vi "LoadAdditionalData.vi"(8 "error in (no error)":errorcluster, 11 "TesteractHAL_DigitalOutput_NIDAQmx In":refnum<class "TesteractHAL_DigitalOutput_NIDAQmx.lvclass">) -> (0 "error out":errorcluster, 3 "TesteractHAL_DigitalOutput_NIDAQmx Out":refnum<class "TesteractHAL_DigitalOutput_NIDAQmx.lvclass">)   [LabVIEW 2017, in "TesteractHAL_DigitalOutput_NIDAQmx.lvlib" / "TesteractHAL_DigitalOutput_NIDAQmx.lvclass"]
doc: "Reads all the data from DeviceCfg and uploads it into the class private data."
uses:
  TesteractHAL_DigitalOutput_NIDAQmx.lvclass
  C:/Program Files (x86)/Testeract/HWLib/HAL/Device/TesteractHAL_Device.lvlibp/TesteractHAL_Device.lvclass
  TesteractHAL_DigitalOutput_NIDAQmx.lvclass/TesteractHAL_DigitalOutput_NIDAQmx.ctl
  Program Files (x86)/Testeract/HWLib/HAL/Device/TesteractHAL_Device.lvlibp/ReadDeviceName.vi
  Program Files (x86)/Testeract/HWLib/HAL/DeviceCfg/TesteractHAL_DeviceCfg_API.lvlibp
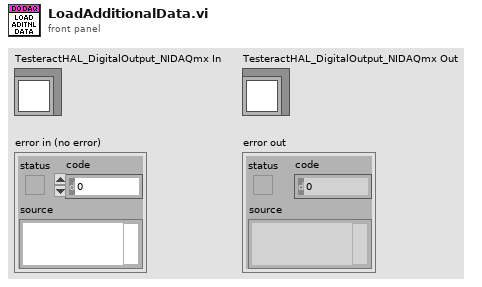
[diagram p1: front panel]
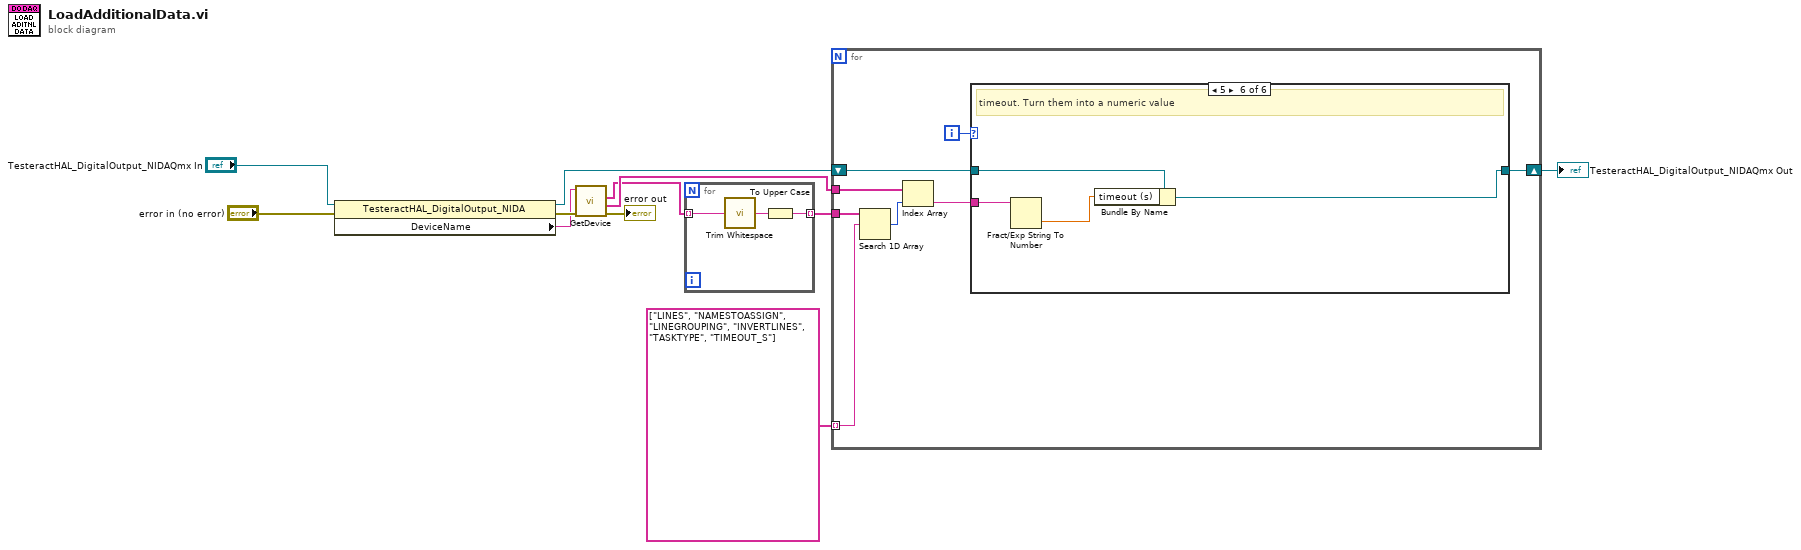
[diagram p0: block diagram]
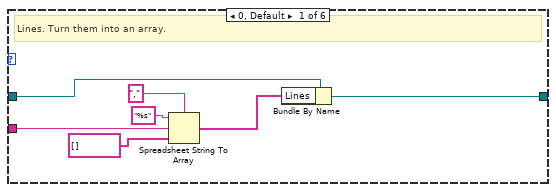
[diagram p2: hidden frame]
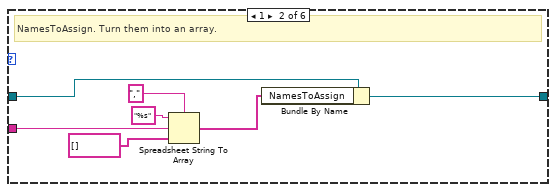
[diagram p3: hidden frame]
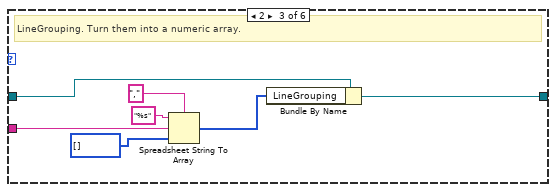
[diagram p4: hidden frame]
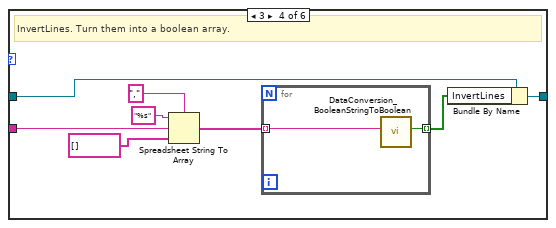
[diagram p5: hidden frame]
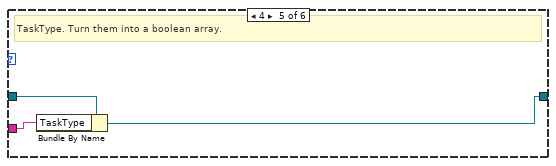
[diagram p6: hidden frame]
diagram:
  n1 = property class="TesteractHAL_DigitalOutput_NIDA"(reference="TesteractHAL_DigitalOutput_NIDAQmx In", error in="error in (no error)") -> (reference out=w2:refnum<class "TesteractHAL_DigitalOutput_NIDAQmx.lvclass">, error out=w9:errorcluster, "DeviceName"=w8:string)
  n2 = call "GetDevice.vi"("error in (no error)"=w9, "Device"=w8) -> ("error out"=→"error out":errorcluster, "Values"=w7:string[], "Keys"=w4:string[])  [unwired: 6 in, 1 out]
  n3 = for {
    tunnel: [w14] -> w5 mode=indexing
    tunnel: w4 -> [w13] mode=indexing
    n4 = call <vilib>:"Trim Whitespace.vi"("string"=w13) -> ("trimmed string"=w12:string)  [unwired: 1 in]
    n5 = To Upper Case(1:w12) -> (0:w14:string)
  }
  n6 = for {
    tunnel: w7 -> [w16]
    tunnel: string[] ["LINES", "NAMESTOASSIGN", "LINEGROUPING", "INVERTLINES", "TASKTYPE", "TIMEOUT_S"] -> [w18] mode=indexing
    tunnel: w5 -> [w17]
    shift-right: [w19] -> w1
    shift-left: w2 -> [w20]
    i -> [w22]
    n7 = Search 1D Array(1D array=w17, element=w18) -> (index of element=w21:i32)  [unwired: 1 in]
    n8 = Index Array(array=w16, index=w21) -> (element=w15:string)
    n9 = case shown="5" w22 {
      tunnel: w20 -> [w29 w35 w42 w50 w55 w59]
      tunnel: [w28 w36 w43 w51 w56 w60] -> w19
      tunnel: w15 -> [w24 w31 w38 w46 w54 w58]
      frame 0, Default {
        # "Lines. Turn them into an array."
        n10 = Spreadsheet String To Array(delimiter (Tab)=",", format string="%s", spreadsheet string=w24, array type (2D Dbl)=string[] []) -> (array=w23:string[])
        n11 = Bundle By Name(cluster=w29, "Lines"=w23) -> (w28:refnum<class "TesteractHAL_DigitalOutput_NIDAQmx.lvclass">)
      }
      frame 1 {
        # "NamesToAssign. Turn them into an array."
        n12 = Spreadsheet String To Array(delimiter (Tab)=",", format string="%s", spreadsheet string=w31, array type (2D Dbl)=string[] []) -> (array=w30:string[])
        n13 = Bundle By Name(cluster=w35, "NamesToAssign"=w30) -> (w36:refnum<class "TesteractHAL_DigitalOutput_NIDAQmx.lvclass">)
      }
      frame 2 {
        # "LineGrouping. Turn them into a numeric array."
        n14 = Spreadsheet String To Array(delimiter (Tab)=",", format string="%s", spreadsheet string=w38, array type (2D Dbl)=i32[] [] ("LineGrouping")) -> (array=w37:i32[])
        n15 = Bundle By Name(cluster=w42, "LineGrouping"=w37) -> (w43:refnum<class "TesteractHAL_DigitalOutput_NIDAQmx.lvclass">)
      }
      frame 3 {
        # "InvertLines. Turn them into a boolean array."
        n16 = Spreadsheet String To Array(delimiter (Tab)=",", format string="%s", spreadsheet string=w46, array type (2D Dbl)=string[] []) -> (array=w45:string[])
        n17 = for {
          tunnel: w45 -> [w53] mode=indexing
          tunnel: [w52] -> w44 mode=indexing
          n18 = call "DataConversion_BooleanStringToBoolean.vi"("Boolean String"=w53) -> ("Boolean Result"=w52:bool)  [unwired: 10 in]
        }
        n19 = Bundle By Name(cluster=w50, "InvertLines"=w44) -> (w51:refnum<class "TesteractHAL_DigitalOutput_NIDAQmx.lvclass">)
      }
      frame 4 {
        # "TaskType. Turn them into a boolean array."
        n20 = Bundle By Name(cluster=w55, "TaskType"=w54) -> (w56:refnum<class "TesteractHAL_DigitalOutput_NIDAQmx.lvclass">)
      }
      frame 5 {
        # "timeout. Turn them into a numeric value"
        n21 = Fract/Exp String To Number(string=w58) -> (number=w57:dbl)  [unwired: 3 in, 1 out]
        n22 = Bundle By Name(cluster=w59, "timeout (s)"=w57) -> (w60:refnum<class "TesteractHAL_DigitalOutput_NIDAQmx.lvclass">)
      }
    }
  }
  "TesteractHAL_DigitalOutput_NIDAQmx Out" <- w1
